vi "Get Wavelength.vi"(8 "error in (no error)":errorcluster, 11 "SpectraPro in":refnum<class "SpectraPro.lvclass">) -> (0 "error out":errorcluster, 2 "Wavelength (nm)":dbl, 3 "SpectraPro out":refnum<class "SpectraPro.lvclass">)   [LabVIEW 2019, in "SpectraPro.lvclass"]
uses:
  SpectraPro.lvclass
  SpectraPro.lvclass/SpectraPro.ctl
  SpectraPro-LabVIEW-Driver/SpectraPro.lvlib
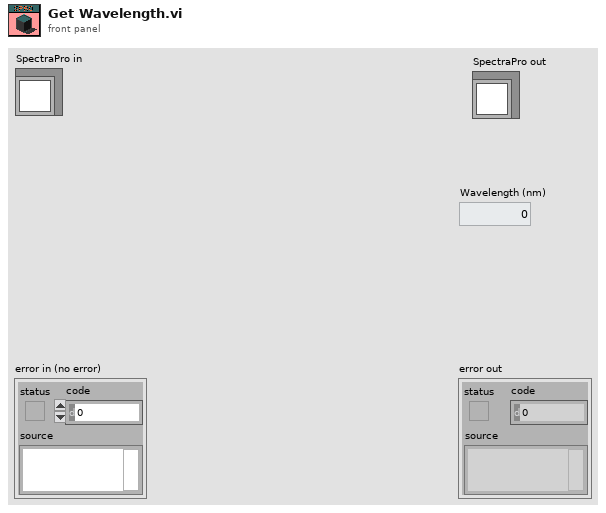
[diagram p1: front panel]
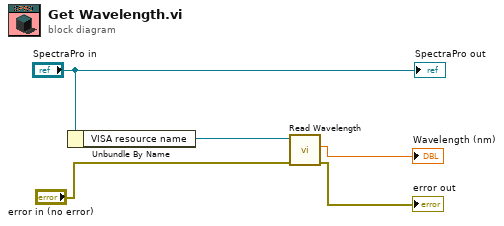
[diagram p0: block diagram]
diagram:
  n1 = Unbundle By Name("SpectraPro in") -> ("VISA resource name"=w2:refnum<visa-resource-name>)
  n2 = call "Read Wavelength.vi"("error in (no error)"="error in (no error)", "VISA resource name"=w2) -> ("error out"=→"error out":errorcluster, "Wavelength (nm)"=→"Wavelength (nm)":dbl)  [unwired: 6 in, 2 out]
  "SpectraPro out" <- "SpectraPro in"
